vi "Calculator.vi"() -> (1 "A 2":string)   [LabVIEW 2018]
panel:
  in  "Enum":enum16{"None", "Divde", "Multi", "Sub", "Add"}(ring)
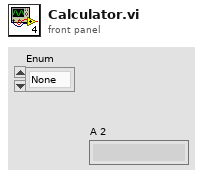
[diagram p1: front panel]
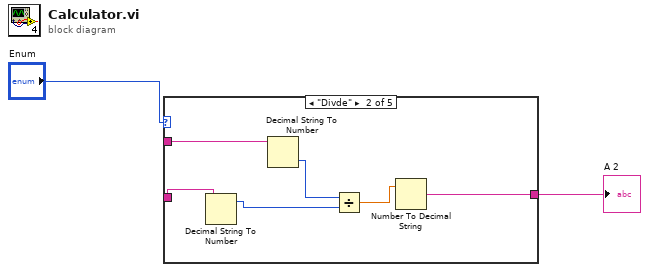
[diagram p0: block diagram]
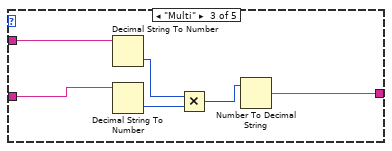
[diagram p3: hidden frame]
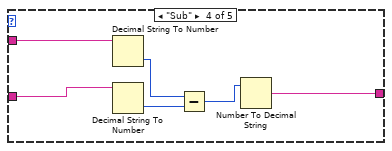
[diagram p4: hidden frame]
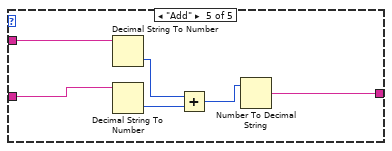
[diagram p5: hidden frame]
diagram:
  n1 = case shown="\"Divde\"" "Enum" {
    tunnel: _ -> [w3 w7 w15 w21 w25]
    tunnel: _ -> [_ w5 w13 w19 w27]
    tunnel: [w3 w9 w10 w16 w22] -> w2
    frame "None", Default {
    }
    frame "Divde" {
      n2 = Decimal String To Number(string=w5) -> (offset past number=w4:i32)  [unwired: 2 in, 1 out]
      n3 = Decimal String To Number(string=w7) -> (number=w6:i32)  [unwired: 2 in, 1 out]
      n4 = Divide(x=w6, y=w4) -> (x/y=w8:dbl)
      n5 = Number To Decimal String(number=w8) -> (decimal integer string=w9:string)  [unwired: 1 in]
    }
    frame "Multi" {
      n6 = Decimal String To Number(string=w15) -> (number=w14:i32)  [unwired: 2 in, 1 out]
      n7 = Decimal String To Number(string=w13) -> (number=w12:i32)  [unwired: 2 in, 1 out]
      n8 = Multiply(x=w14, y=w12) -> (x*y=w11:i32)
      n9 = Number To Decimal String(number=w11) -> (decimal integer string=w10:string)  [unwired: 1 in]
    }
    frame "Sub" {
      n10 = Decimal String To Number(string=w21) -> (number=w20:i32)  [unwired: 2 in, 1 out]
      n11 = Decimal String To Number(string=w19) -> (number=w18:i32)  [unwired: 2 in, 1 out]
      n12 = Subtract(x=w20, y=w18) -> (x-y=w17:i32)
      n13 = Number To Decimal String(number=w17) -> (decimal integer string=w16:string)  [unwired: 1 in]
    }
    frame "Add" {
      n14 = Decimal String To Number(string=w25) -> (number=w24:i32)  [unwired: 2 in, 1 out]
      n15 = Decimal String To Number(string=w27) -> (number=w26:i32)  [unwired: 2 in, 1 out]
      n16 = Add(x=w24, y=w26) -> (x+y=w23:i32)
      n17 = Number To Decimal String(number=w23) -> (decimal integer string=w22:string)  [unwired: 1 in]
    }
  }
  "A 2" <- w2
